vi "Motors.vi"(7 "x":i32, 8 "error in (no error)":errorcluster, 9 "VelValIn":dbl[](array[numeric])=[0.0, 0.0, 0.0], 10 "steering frame in":refnum<class "NI_Robotics_Steering Frame.lvclass">, 11 "FPGA VI Reference In":refnum<k20>) -> (0 "error out":errorcluster, 1 "VAL":dbl[](array[numeric]), 2 "steering frame out":refnum<class "NI_Robotics_Steering Frame.lvclass">, 3 "FPGA VI Reference  out":refnum<k20>)   [LabVIEW 2019]
uses:
  <vilib>/robotics/Steering/Steering Frame/NI_Robotics_Steering Frame.lvclass
  <vilib>/Utility/error.llb/Error Cluster From Error Code.vi
  <vilib>/rvi/errors/niLvFpgaAdjustHostInterfaceError.vi
  <vilib>/rvi/interface/nirviReadWriteControl/nirviReadWriteControl.xnode
  NiFpgaLv.dll
  <vilib>/rvi/interface/Simulation/niFpgaSimulationCallBeginRW.vi
panel:
  out "Destination":dbl[](array[numeric])
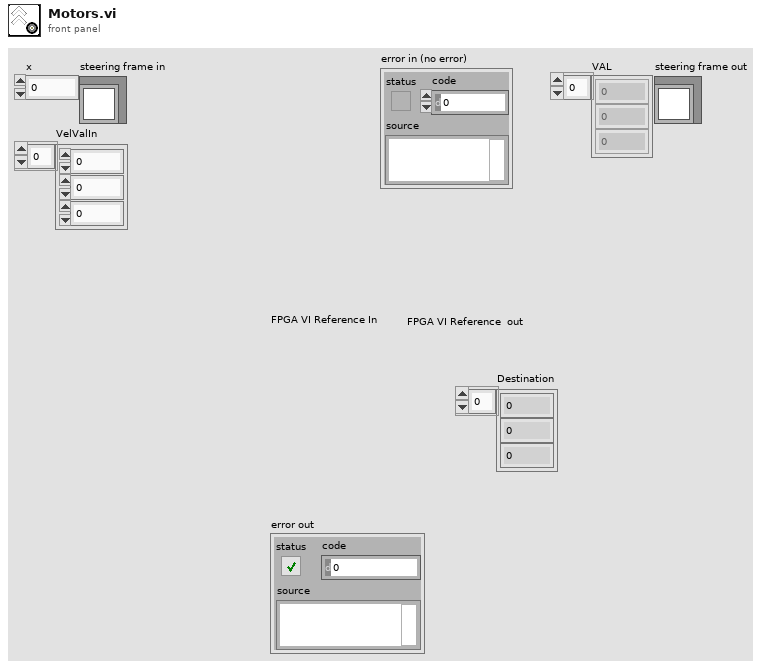
[diagram p1: front panel]
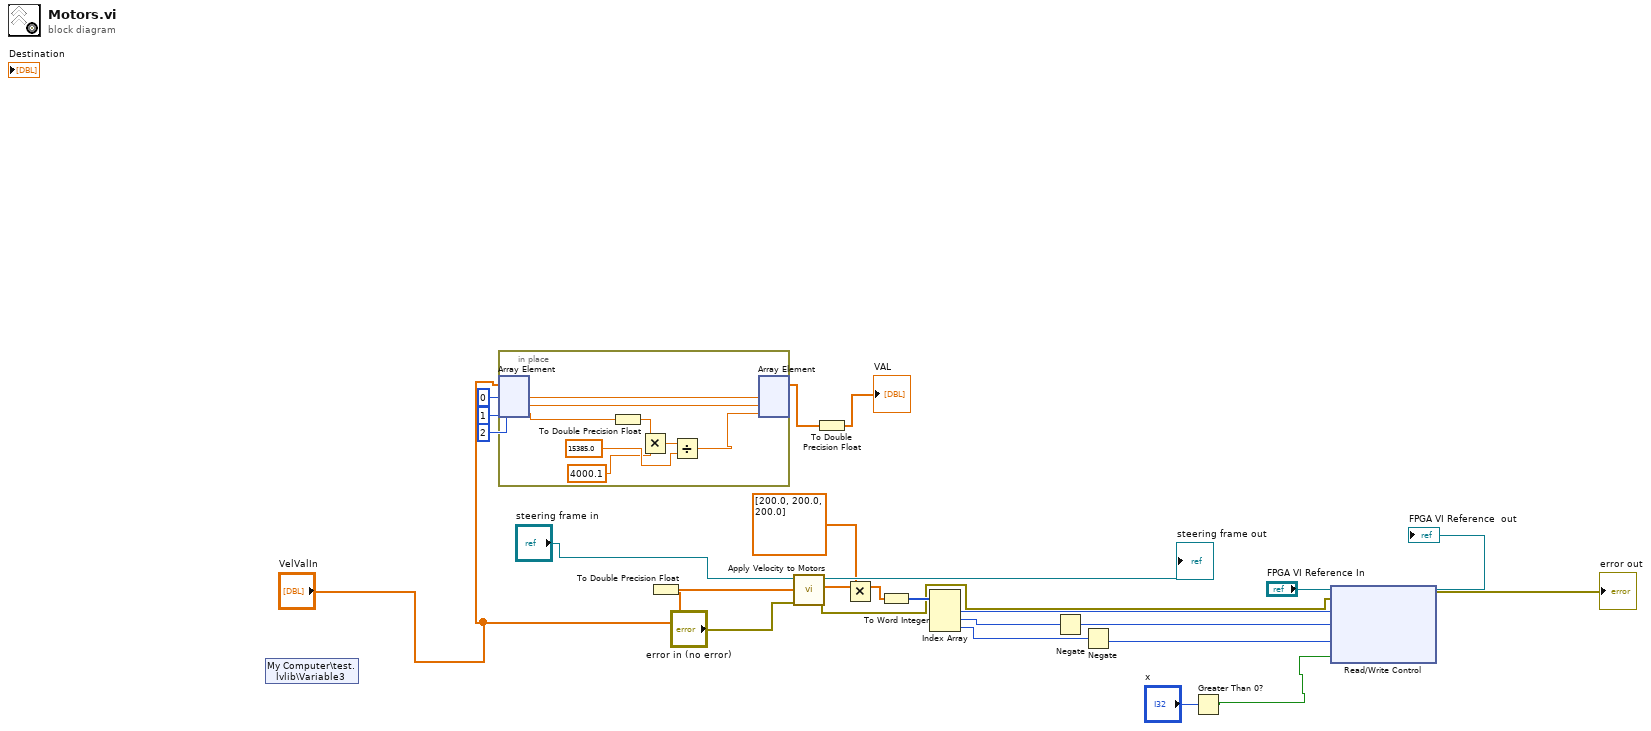
[diagram p0: block diagram]
diagram:
  n1 = shared-variable "My Computer\\test.lvlib\\Variable3"() -> ()  [unwired: 1 in, 2 out]
  n2 = in-place {
    n3 = in-place-array #1("VelValIn", 0, 1, 2) -> (w33:dbl, w32:dbl, w27:dbl)
    n4 = To Double Precision Float(number=w27) -> (double precision float=w26:dbl)
    n5 = Multiply(x=w26, y=4000.1) -> (x*y=w31:dbl)
    n6 = Divide(x=w31, y=15385.0) -> (x/y=w28:dbl)
    n7 = in-place-array #1(w33, w32, w28) -> (w4:dbl[])  [unwired: 3 out]
  }
  n8 = To Double Precision Float(number="VelValIn") -> (double precision float=w2:dbl[])
  n9 = call-poly <vilib>:"Apply Velocity to Motors.vi"("error in (no error)"="error in (no error)", "steering frame velocity"=w2, "steering frame in"="steering frame in") -> ("error out"=w13:errorcluster, "ccw motor velocity setpoints"=w24:dbl[], "steering frame out"=→"steering frame out":refnum<class "NI_Robotics_Steering Frame.lvclass">)  [unwired: 4 in, 2 out]
  n10 = To Double Precision Float(number=w4) -> (double precision float=→"VAL":dbl[])
  n11 = Multiply(x=w24, y=dbl[] [200.0, 200.0, 200.0]) -> (x*y=w6:dbl[])
  n12 = To Word Integer(number=w6) -> (16bit integer=w19:i16[])
  n13 = Index Array(array=w19) -> (element #1=w23:i16, element #2=w20:i16, element #3=w21:i16)  [unwired: 3 in]
  n14 = Negate(x=w20) -> (-x=w18:i16)
  n15 = Negate(x=w21) -> (-x=w22:i16)
  n16 = Greater Than 0?(x="x") -> (x > 0?=w8:bool)
  n17 = xnode "Read/Write Control"("FPGA VI Reference In"="FPGA VI Reference In", "error in"=w13, "M1"=w23, "M2"=w18, "M3"=w22, "RESET ENCODER"=w8) -> ("FPGA VI Reference Out"=→"FPGA VI Reference  out":refnum<k20>, "error out"=→"error out":errorcluster)
